vi "InitializeLaser.vi"(8 "error in":errorcluster, 10 "ON/OFF":bool, 11 "VISA resource name in":refnum<visa-resource-name>) -> (0 "error out":errorcluster, 3 "VISA resource name out":refnum<visa-resource-name>, 4 "Tmax":dbl, 5 "SN:":string, 6 "Tmin":dbl, 7 "Лазер: ID:":string)   [LabVIEW 2014]
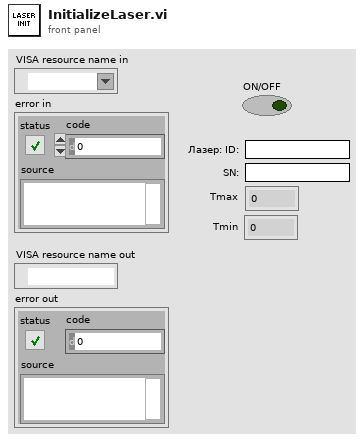
[diagram p1: front panel]
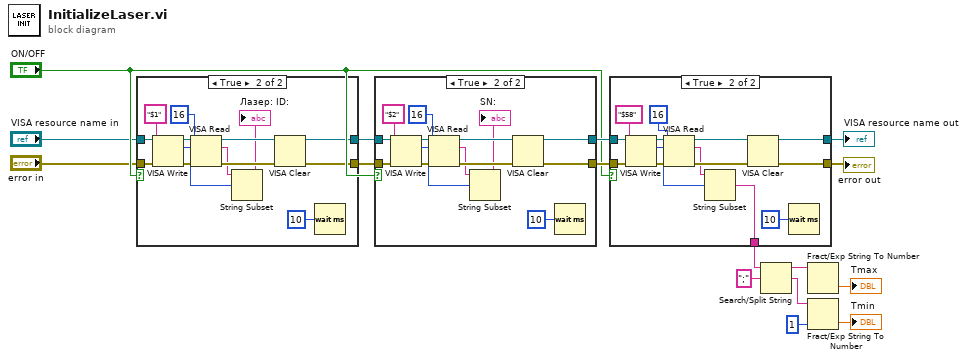
[diagram p0: block diagram]
diagram:
  n1 = case shown="True" "ON/OFF" {
    tunnel: "VISA resource name in" -> [w18 w30]
    tunnel: "error in" -> [w17 w29]
    tunnel: [w18 w25] -> w12
    tunnel: [w17 w24] -> w11
    frame False {
    }
    frame True {
      n2 = VISA Write(VISA resource name=w30, write buffer="$1", error in (no error)=w29) -> (VISA resource name out=w31:refnum<visa-resource-name>, return count=w21:u32, error out=w32:errorcluster)
      n3 = VISA Read(VISA resource name=w31, byte count=u32 16, error in (no error)=w32) -> (VISA resource name out=w27:refnum<visa-resource-name>, read buffer=w19:string, error out=w26:errorcluster)  [unwired: 1 out]
      n4 = String Subset(string=w19, offset (0)=w21) -> (substring=→"Лазер: ID:":string)  [unwired: 1 in]
      n5 = VISA Clear(VISA resource name=w27, error in (no error)=w26) -> (VISA resource name out=w25:refnum<visa-resource-name>, error out=w24:errorcluster)
      n6 = Wait (ms)(milliseconds to wait=u32 10) -> ()  [unwired: 1 out]
    }
  }
  n7 = case shown="True" "ON/OFF" {
    tunnel: w12 -> [w34 w46]
    tunnel: w11 -> [w33 w45]
    tunnel: [w34 w41] -> w10
    tunnel: [w33 w40] -> w9
    frame False {
    }
    frame True {
      n8 = VISA Write(VISA resource name=w46, write buffer="$2", error in (no error)=w45) -> (VISA resource name out=w47:refnum<visa-resource-name>, return count=w37:u32, error out=w48:errorcluster)
      n9 = VISA Read(VISA resource name=w47, byte count=u32 16, error in (no error)=w48) -> (VISA resource name out=w43:refnum<visa-resource-name>, read buffer=w36:string, error out=w42:errorcluster)  [unwired: 1 out]
      n10 = String Subset(string=w36, offset (0)=w37) -> (substring=→"SN:":string)  [unwired: 1 in]
      n11 = VISA Clear(VISA resource name=w43, error in (no error)=w42) -> (VISA resource name out=w41:refnum<visa-resource-name>, error out=w40:errorcluster)
      n12 = Wait (ms)(milliseconds to wait=u32 10) -> ()  [unwired: 1 out]
    }
  }
  n13 = case shown="True" "ON/OFF" {
    tunnel: w10 -> [w50 w62]
    tunnel: w9 -> [w49 w61]
    tunnel: [w50 w57] -> w2
    tunnel: [w49 w56] -> w1
    tunnel: [_ w53] -> w8
    frame False {
    }
    frame True {
      n14 = VISA Write(VISA resource name=w62, write buffer="$58", error in (no error)=w61) -> (VISA resource name out=w63:refnum<visa-resource-name>, return count=w52:u32, error out=w64:errorcluster)
      n15 = VISA Read(VISA resource name=w63, byte count=u32 16, error in (no error)=w64) -> (VISA resource name out=w59:refnum<visa-resource-name>, read buffer=w51:string, error out=w58:errorcluster)  [unwired: 1 out]
      n16 = String Subset(string=w51, offset (0)=w52) -> (substring=w53:string)  [unwired: 1 in]
      n17 = VISA Clear(VISA resource name=w59, error in (no error)=w58) -> (VISA resource name out=w57:refnum<visa-resource-name>, error out=w56:errorcluster)
      n18 = Wait (ms)(milliseconds to wait=u32 10) -> ()  [unwired: 1 out]
    }
  }
  "VISA resource name out" <- w2
  "error out" <- w1
  n19 = Search/Split String(string=w8, search string/char (-)=";") -> (substring before match=w15:string, match + rest of string=w14:string)  [unwired: 1 in, 1 out]
  n20 = Fract/Exp String To Number(string=w15) -> (number=→"Tmax":dbl)  [unwired: 3 in, 1 out]
  n21 = Fract/Exp String To Number(string=w14, offset=1) -> (number=→"Tmin":dbl)  [unwired: 2 in, 1 out]
